vi "Dashboard Main.vi"() -> ()   [LabVIEW 2018]
uses:
  <vilib>/Utility/miscctls.llb/LVRowAndColumnTypeDef.ctl
  <vilib>/event_ctls.llb/eventvkey.ctl
  <vilib>/Rock Robotics/Network Tables/NT Read Numeric Array.vi
  <vilib>/Rock Robotics/Network Tables/NT Write Boolean.vi
  <vilib>/Rock Robotics/WPI/Dashboard/WPI_DashboardLogging Global.vi
panel:
  in  "Camera Settings Right":T1={"Frame Rate"=30, "Compression"=30, "Size"=1, "DB Camera Config"=FALSE} {"Frame Rate" scale=1.0..30.0; "Compression" scale=100.0..-1.0; "Size" items=["640x480", "320x240", "160x120"]}
  in  "Camera Name Right":string(combo)="No Camera Selection"
  out "Camera Perf":string
  in  "Camera Settings":T1={"Frame Rate"=30, "Compression"=30, "Size"=1, "DB Camera Config"=FALSE} {"Frame Rate" scale=1.0..30.0; "Compression" scale=100.0..-1.0; "Size" items=["640x480", "320x240", "160x120"]}
  in  "TCP":refnum<k5>
  in  "Rec Mode":enum32{"Stop", "Record", "Playback"}(radio)
  out "Robot IP":string
  out "Image Message":string="Timeout in Camera Communications"
  in  "Dashboard Tab":T2(tab)
  in  "Select Auto":string(combo)="Select Autonomous ..."
  out "NT Connection":bool
  out "MotorChart R":cluster{"Numeric":dbl, "Numeric":dbl}(graph)
  out "MotorChart L":cluster{"Numeric":dbl, "Numeric":dbl}(graph)
  out "MotorSliders R":cluster{"MotorSlide1":dbl, "MotorSlide2":dbl} {"MotorSlide2" scale=-1.0..1.0 scale format="%#_2e"; "MotorSlide1" scale=-1.0..1.0 scale format="%#_2e"}
  out "MotorSliders L":cluster{"MotorSlide1":dbl, "MotorSlide2":dbl} {"MotorSlide2" scale=-1.0..1.0 scale format="%#_2e"; "MotorSlide1" scale=-1.0..1.0 scale format="%#_2e"}
  out "Gyro":dbl(knob) scale=0.0..360.0
  out "JS1 Z":dbl(slide) scale=-1.0..1.0 scale format="%#_2e"
  out "JS1 Graph":cluster{"X":dbl, "Y":dbl}[](graph)
  out "JS1 Buttons":T3
  out "JS2 Z":dbl(slide) scale=-1.0..1.0 scale format="%#_2e"
  out "JS2 Graph":cluster{"X":dbl, "Y":dbl}[](graph)
  out "JS2 Buttons":T3
  out "Mode":T4(ring)=enum."Auto Disabled"
  out "Right Camera Perf":cluster{"Bandwidth (Mbps)":dbl, "FPS":dbl}
  out "Camera Image Right":T5(plugin-control)
  in  "DB/String 9":string
  in  "DB/String 8":string
  in  "DB/String 7":string
  in  "DB/String 6":string
  in  "DB/String 5":string
  in  "DB/String 4":string
  in  "DB/String 3":string
  in  "DB/String 2":string
  in  "DB/String 1":string
  in  "DB/String 0":string
  in  "DB/Slider 0":dbl(slide) scale=0.0..5.0
  in  "DB/Slider 1":dbl(slide) scale=0.0..5.0
  in  "DB/Slider 2":dbl(slide) scale=0.0..5.0
  in  "DB/Slider 3":dbl(slide) scale=0.0..5.0
  out "DB/LED 3":bool
  out "DB/LED 2":bool
  out "DB/LED 1":bool
  out "DB/LED 0":bool
  in  "DB/Button 3":bool
  in  "DB/Button 2":bool
  in  "DB/Button 1":bool
  in  "DB/Button 0":bool caption="New Name"
  in  "Mode":T6(ring)
  in  "Zero Horse Encoder":bool
  in  "Zero Elevator Encoder":bool
  in  "Zero Wrist Encoder":bool
  in  "Place Level 3":bool
  in  "Place Level 2":bool
  in  "Place Level 1":bool
  in  "Cargo Ship":bool
  in  "Intake Feeder":bool
  in  "Intake Ground":bool
  in  "Elevator Control":dbl(slide) step=0.05 scale=-1.0..1.0
  in  "Wrist Control":dbl(slide) step=0.05 scale=-1.0..1.0
  in  "Test Slider":dbl(slide) scale=0.0..100.0 scale format="%#_3g"
  in  "On/Off":bool caption="Solenoid"
  in  "Test Name":u16(ring) items=["Select the test to run..."]
  in  "Test Tree":string(tree)
  in  "Motor":cluster{"Value":dbl, "Enable":bool} {"Value" scale=-1.0..1.0 scale format="%#_3g"}
  out "Progress":T7 {"Test Progress" scale=0.0..100.0}
  in  "Rev/Fwd":cluster{"Forward":bool, "Reverse":bool}
  in  "Test Ring":u16(ring) items=["Monochrome", "Color"]
  out "Cmd Status":string
  in  "Execute Command":bool
  in  "Command Params":string[][](table)
  in  "Command Selection":i32(listbox)
  in  "CheckList":i32(listbox)
  out "Tree":string(tree)
  out "Camera Image":T5(plugin-control)
  out "Background":bool
  in  "Camera Name":string(combo)="No Camera Selection"
  # "HW"
  # "HW"
  # "Joysticks"
  # "Drive Motors"
  # "Front"
  # "Right"
  # "Left"
  # "Back"
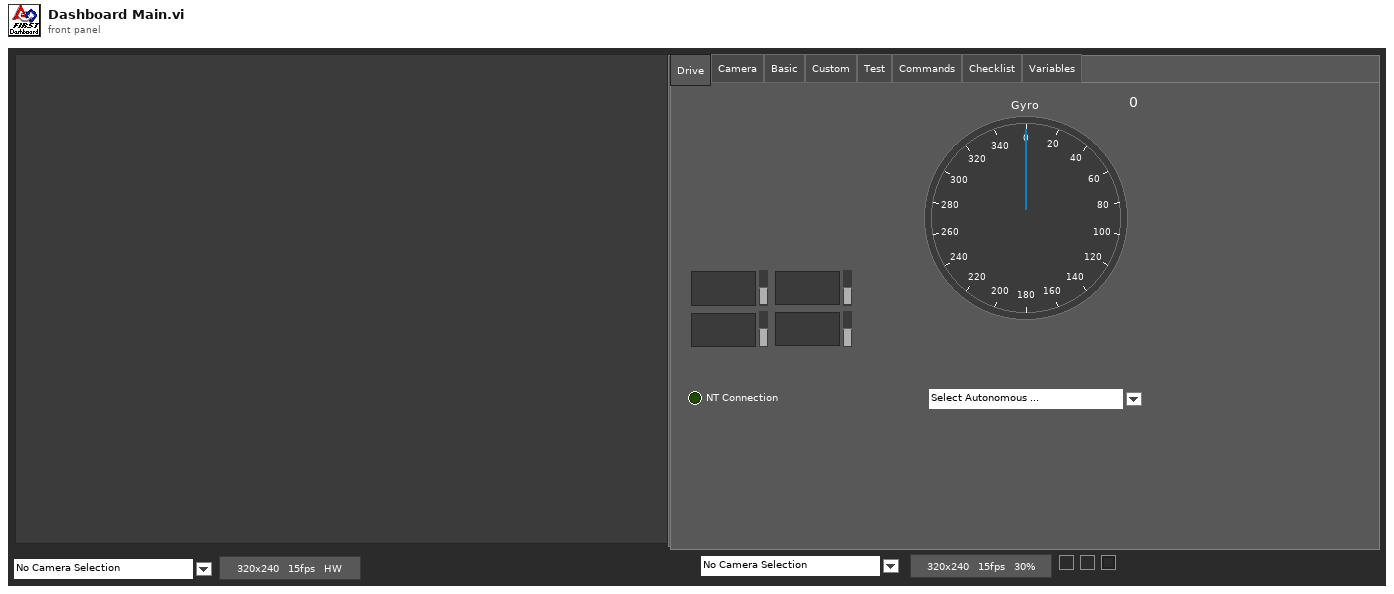
[diagram p1: front panel]
types:
  T1 = cluster{"Frame Rate":i32, "Compression":i32, "Size":u16, "DB Camera Config":bool}
  T2 = enum32{"Drive", "Camera", "Basic", "Custom", "Test", "Commands", "Checklist", "Variables"}
  T3 = cluster{bool, bool, bool, bool, bool, bool, bool, bool, bool, bool, bool, bool}
  T4 = enum8{"Tele-Op Disabled", "Tele-Op Enabled", "Auto Disabled", "Auto Enabled", "Test Disabled", "Test Enabled", "Disconnected", "No Code", "E-Stop"}
  T5 = typedef "IMAQ Image.ctl" = refnum<image>
  T6 = enum16{"Operator Console", "Hatch", "Cargo", "Horse Hatch", "Override to Manual"}
  T7 = cluster{"Test Progress":u8, "Test Progress Text":string}
  T8 = cluster{"Save Path":path, "Interval (s)":dbl, "Keep":i32}
  T9 = typedef "Image Type" = u32
  T10 = cluster{"IDs":cluster{"RPC field ID":u16, "Unique ID":u16}, "String":string}
  T11 = cluster{"Error Strings":string, "Disable Counts":cluster{u16, u16}, "Rail Faults":cluster{u16, u16, u16}, "Robot IP":string, "DB Mode":u8, "Event Info":cluster{"Name":string, "Type":u8, "Number":u16, "Replay":u8}}
  T12 = cluster{"Storage":cluster{"Disk Free":u64, "RAM Block":u32, "RAM free":u32}, "CPU Utilization":cluster{"CPU % ISR":sgl, "CPU % Time Crit":sgl, "CPU % Timed Str":sgl, "CPU % High":sgl, "CPU % Above":sgl, "CPU % Normal":sgl, "CPU % Low":sgl}, "CAN":cluster{"% Bus Utilization":sgl, "Bus Off Cnt":u32, "TX_FIFO Full Cnt":u32, "Receive Error Cnt":u8, "Transmit Error Cnt":u8}, "HID":cluster{"HID Outputs":u32, "Rumble Low":u16, "Rumble High":u16}[]}
  T13 = cluster{"Status bits":cluster{"Test Mode":bool, "Autonomous":bool, "Enabled":bool, "Code Start":bool, "Brownout":bool, "Reserved 2":bool, "Reserved 3":bool, "E-Stop":bool}, "Code Trace":cluster{"Disabled":bool, "TeleOp":bool, "Auto":bool, "Test":bool}, "Controller Type":enum16{"unknown", "cRIO", "roboRio"}, "Code?":enum16{"unknown", "noCode", "code"}, "Battery V":dbl}
  T14 = cluster{"Control Bits":cluster{"TestMode":bool, "Autonomous":bool, "Enabled":bool, "FMS Present":bool, bool, bool, bool, "E-Stop":bool}, "Team Station ":u8, "Countdown":sgl, "Joystick Values":cluster{"Axes":dbl[], "Buttons":bool[], "POVs":i16[]}[]}
  T15 = cluster{"Axes":dbl[], "Buttons":bool[], "POVs":i16[]}[]
  T16 = cluster{"Axes":dbl[], "Buttons":bool[], "POVs":i16[]}
  T17 = cluster{"Buttons[0]":bool, "Buttons[1]":bool, "Buttons[2]":bool, "Buttons[3]":bool, "Buttons[4]":bool, "Buttons[5]":bool, "Buttons[6]":bool, "Buttons[7]":bool, "Buttons[8]":bool, "Buttons[9]":bool, "Buttons[10]":bool, "Buttons[11]":bool}
  T18 = cluster{"Camera Image":refnum<vi>, "Dashboard Tab":refnum<vi>, "Background":refnum<vi>, "Rec Mode":refnum<vi>, "Test Slider":refnum<vi>, "On/Off ":refnum<vi>, "Test Ring":refnum<vi>, "Rev/Fwd":refnum<vi>, "Test Name":refnum<vi>, "Motor":refnum<vi>, "Progress":refnum<vi>, "CheckList":refnum<vi>, "Tree":refnum<vi>, "Test Tree":refnum<vi>, "Command Params":refnum<vi>, "Command Selection":refnum<vi>, "Execute Command":refnum<vi>, "Cmd Status":refnum<vi>, "Camera Settings":refnum<vi>, "Camera Name":refnum<vi>, "Camera Perf":refnum<vi>, "Camera Settings Right":refnum<vi>, "Camera Name Right":refnum<vi>, "Camera Image Right":refnum<vi>}
  T19 = cluster{"Global Rectangle":i32[], "Contours":cluster{"Contour Type":u32, "ROI Type":u32, "Points":i32[]}[]}
  T20 = cluster{"Camera Name":string, string, "Saved DB Images Info":cluster{"Save Path":path, "Interval (s)":dbl, "Keep":i32}}
  T21 = cluster{"Camera Name Right":string, string, "Saved DB Images Info":cluster{"Save Path":path, "Interval (s)":dbl, "Keep":i32}}
  T22 = cluster{"Operation":enum16{"Update", "Clear"}, "Color Box":u32}[]
  T23 = typedef "eventvkey.ctl" = enum16{"ASCII", "Enter", "Return", "Shift", "Ctrl", "Alt", "Cmd", "Opt", "Caps", "NumLock", "Clear", "Break", "Up", "Down", "Left", "Right", "Insert", "Delete", "Home", "End", "PageUp", "PageDown", "Escape", "Help", "Pause", "ScrollLock", "F1", "F2", "F3", "F4", "F5", "F6", "F7", "F8", "F9", "F10", "F11", "F12", "F13", "F14", "F15", "F16", "F17", "F18", "F19", "F20", "F21", "F22", "F23", "F24", "Play", "VolumeUp", "VolumeDown", "Mute", "Two Byte Char"}
  T24 = cluster{"Image Size":bool, "Image Type":bool, "Pixel Value":bool, "ROI Information":bool, "Zoom Factor":bool}
  T25 = cluster{"Operation":enum16{"Update", "Clear"}, "Color Box":u32}
  T26 = typedef "LVRowAndColumnTypeDef.ctl" = cluster{"Row":i32, "Column":i32}
  T27 = cluster{"Shift":bool, "Ctrl":bool, "Alt":bool, "Cmd":bool, "Opt":bool}
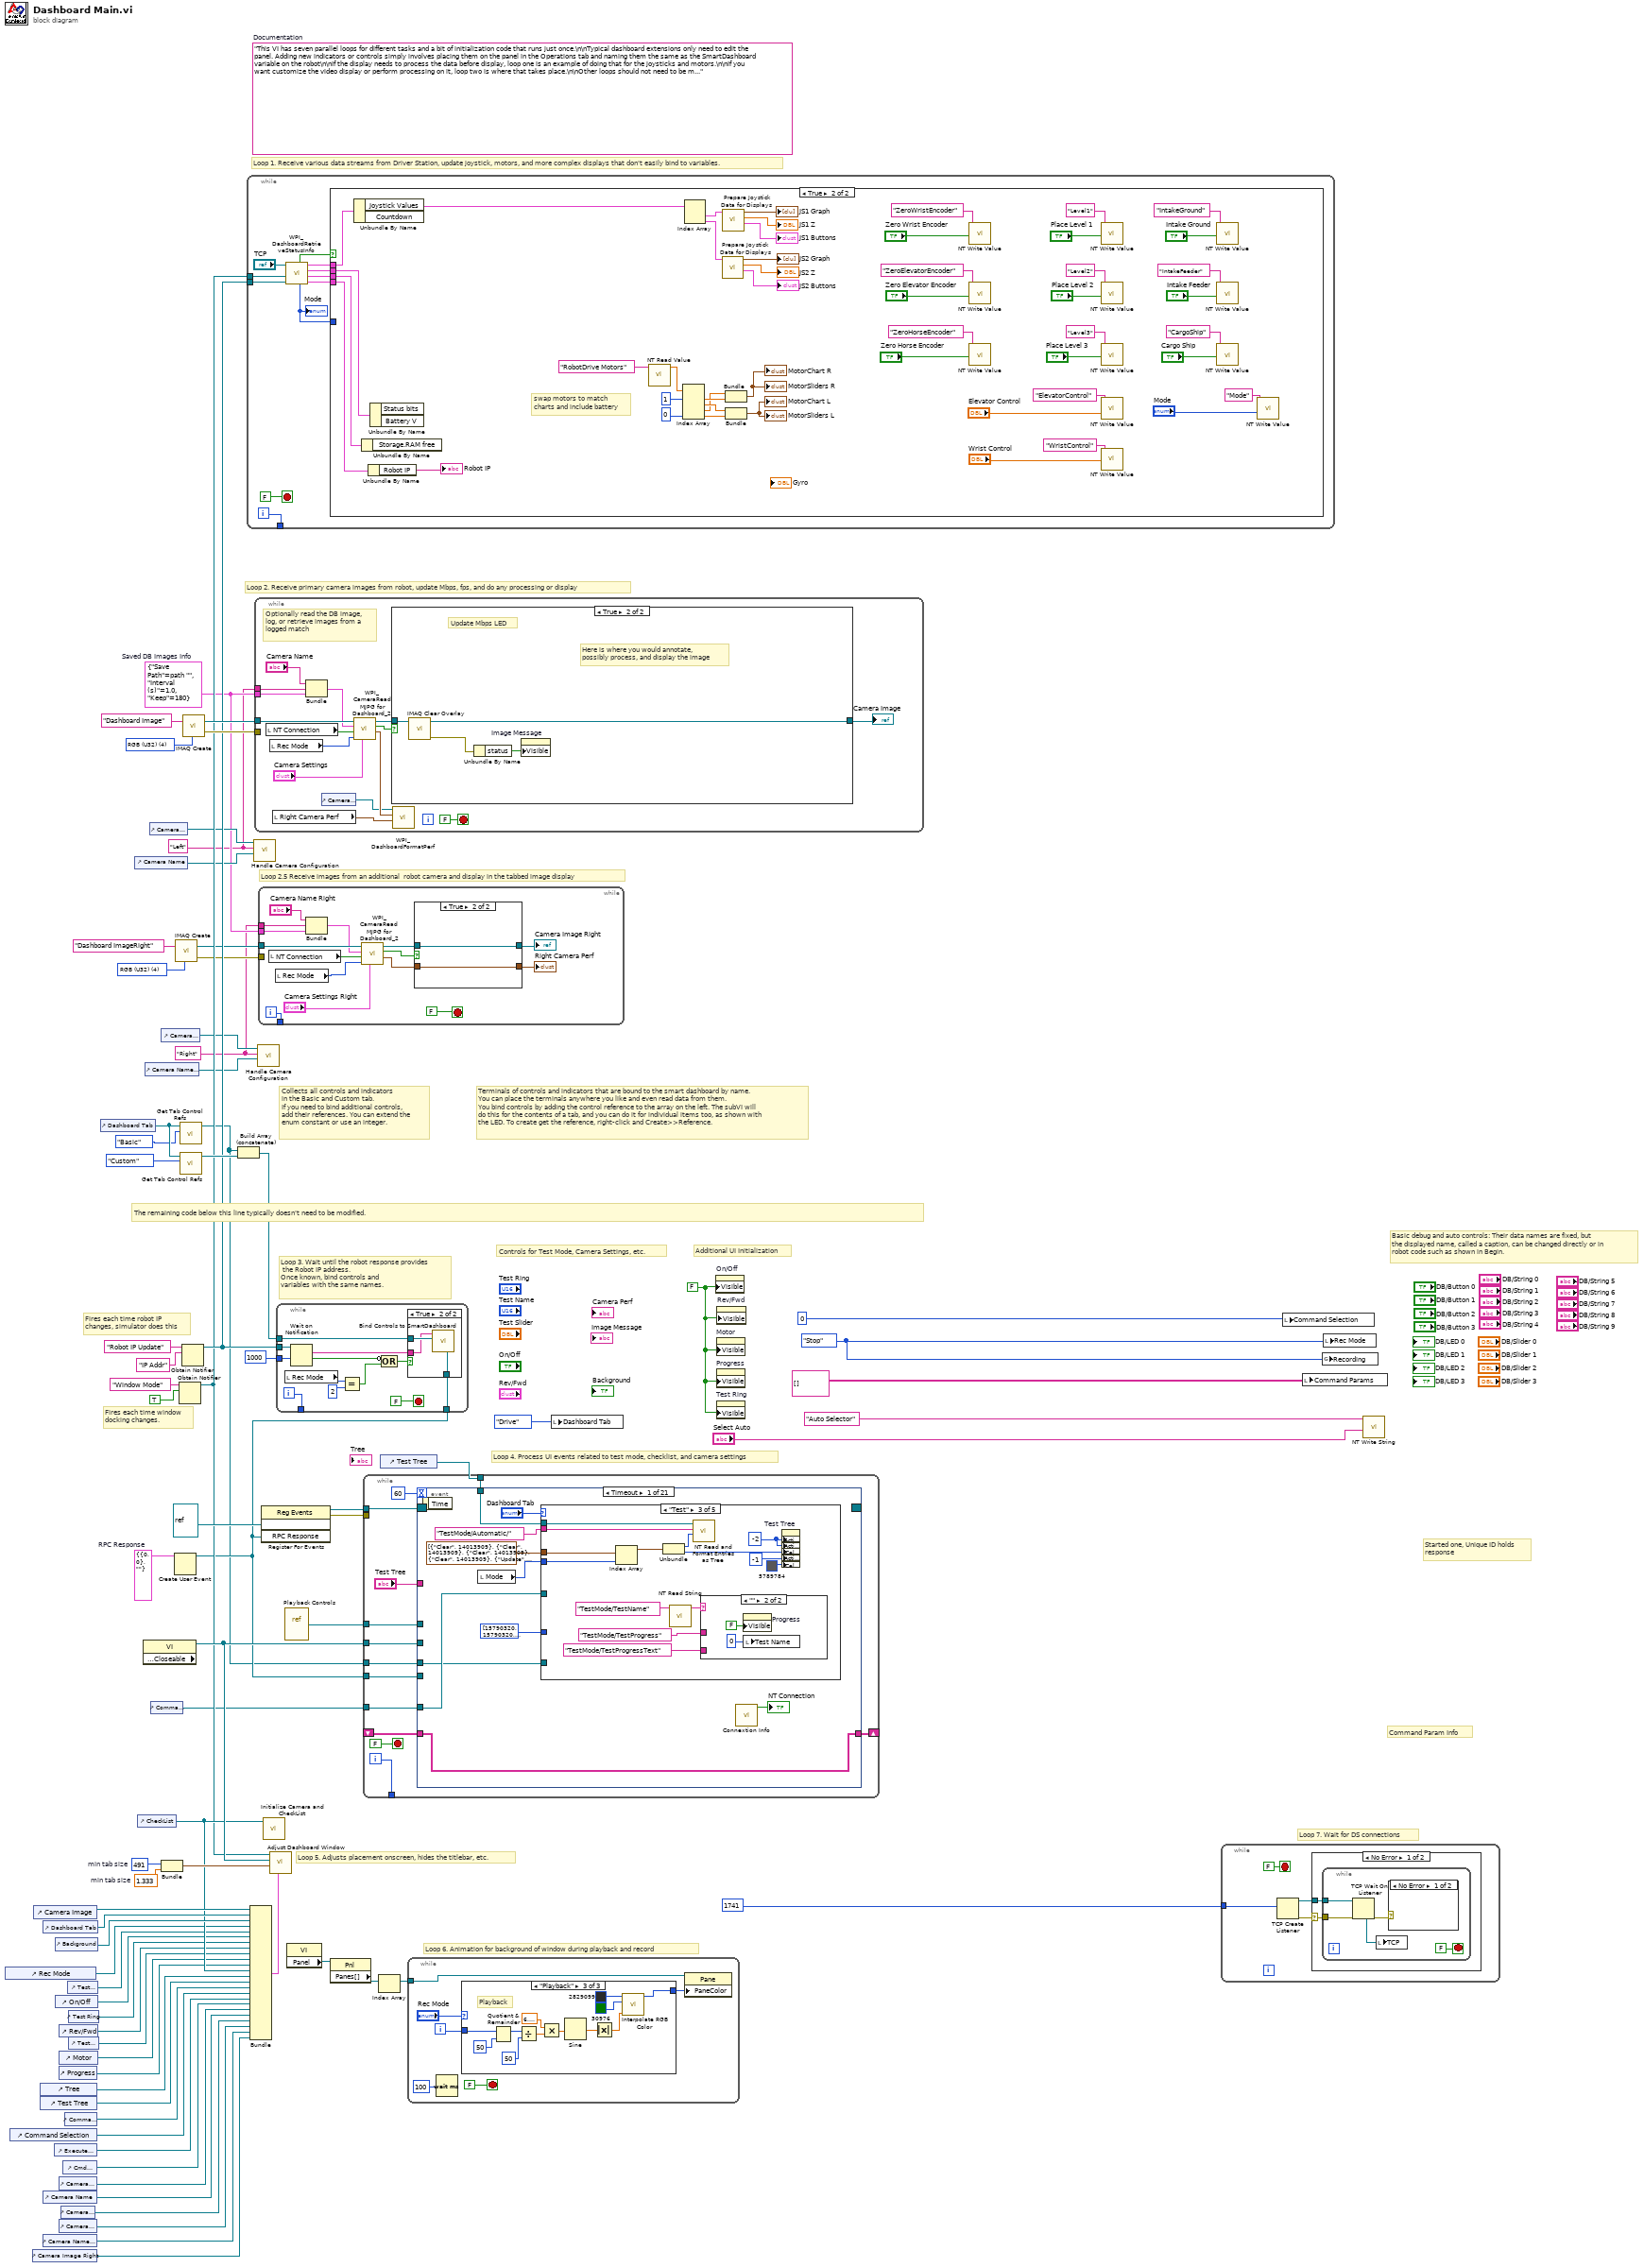
[diagram p0: block diagram]
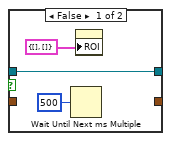
[diagram p2: hidden frame]
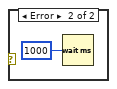
[diagram p3: hidden frame]
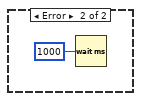
[diagram p4: hidden frame]
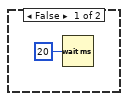
[diagram p5: hidden frame]
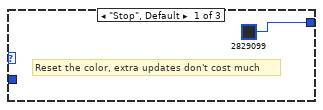
[diagram p6: hidden frame]
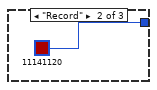
[diagram p7: hidden frame]
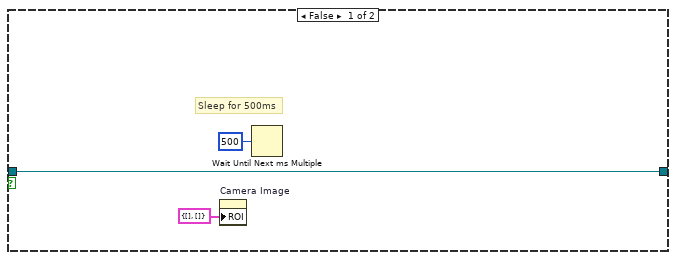
[diagram p9: hidden frame]
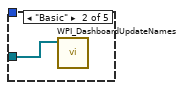
[diagram p11: hidden frame]
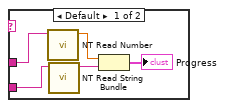
[diagram p12: hidden frame]
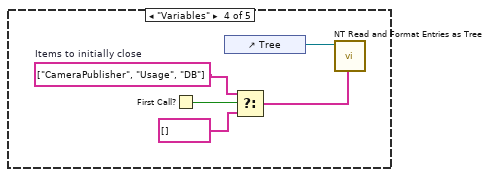
[diagram p13: hidden frame]
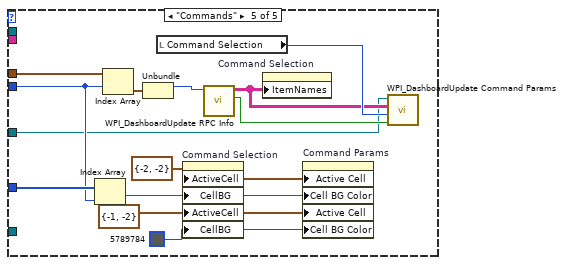
[diagram p14: hidden frame]
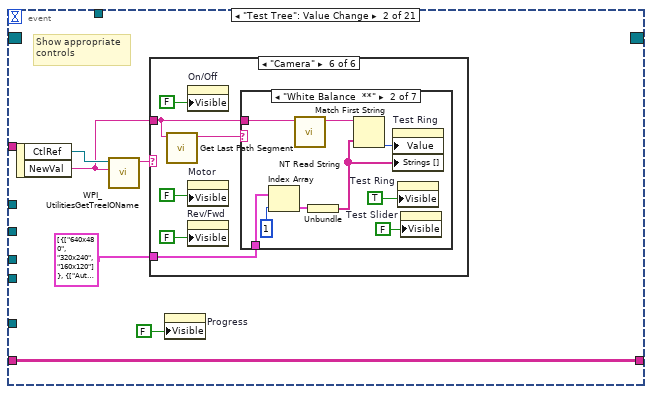
[diagram p15: hidden frame]
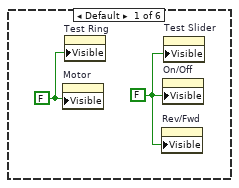
[diagram p16: hidden frame]
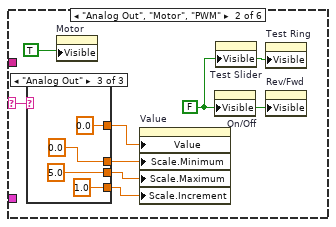
[diagram p17: hidden frame]
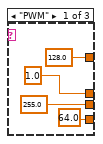
[diagram p18: hidden frame]
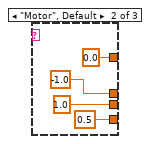
[diagram p19: hidden frame]
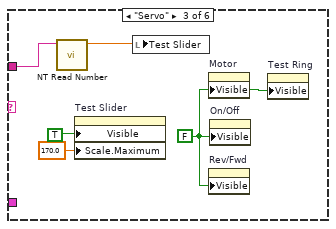
[diagram p20: hidden frame]
diagram:
  w3 = T8 {"Save Path"=path "", "Interval (s)"=1.0, "Keep"=180}  # Saved DB Images Info
  w2 = "Right"
  w1 = "Left"
  w13 = T9 4 items=["Grayscale (U8)", "Grayscale (I16)", "Grayscale (SGL)", "Complex (CSG)", "RGB (U32)", "HSL (U32)", "RGB (U64)"] ("Image Type")
  w29 = T10 {"IDs"={"RPC field ID"=0, "Unique ID"=0}, "String"=""}  # RPC Response
  w52 = 491  # min tab size
  w51 = 1.333  # min tab size
  w59 = enum32{"Stop", "Record", "Playback"}."Stop" ("Rec Mode")
  w36 = FALSE ("Visible")
  (unwired) "This VI has seven parallel loops for different tasks and a bit of initialization code that runs just once.\n\nTypical dashboard extensions only need to edit the panel. Adding new indicators or controls simply involves placing them on the panel in the Operations tab and naming them the same as the SmartDashboard variable on the robot\n\nIf the display needs to process the data before display, loop one is an example of doing that for the joysticks and motors.\n\nIf you want customize the video display or perform processing on it, loop two is where that takes place.\n\nOther loops should not need to be modified. They are pretty standard, and document the task they perform."  # Documentation
  w76 = T9 4 items=["Grayscale (U8)", "Grayscale (I16)", "Grayscale (SGL)", "Complex (CSG)", "RGB (U32)", "HSL (U32)", "RGB (U64)"] ("Image Type")
  # "Loop 2.5 Receive images from an additional  robot camera and display in the tabbed image display"
  # "Command Param Info"
  # "Started one, Unique ID holds\nresponse"
  # "Loop 7. Wait for DS connections"
  # "Basic debug and auto controls: Their data names are fixed, but\nthe displayed name, called a caption, can be changed directly or in\nrobot code such as shown in Begin."
  # "Controls for Test Mode, Camera Settings, etc."
  # "Additional UI Initialization"
  # "Loop 6. Animation for background of window during playback and record"
  # "Fires each time robot IP\nchanges, simulator does this"
  # "Fires each time window\ndocking changes."
  # "Collects all controls and indicators\nin the Basic and Custom tab.\nIf you need to bind additional controls,\nadd their references. You can extend the\nenum constant or use an integer."
  # "The remaining code below this line typically doesn't need to be modified."
  # "Loop 4. Process UI events related to test mode, checklist, and camera settings"
  # "Terminals of controls and indicators that are bound to the smart dashboard by name.\nYou can place the terminals anywhere you like and even read data from them.\nYou bind controls by adding the control reference to the array on the left. The subVI will\ndo this for the contents of a tab, and you can do it for individual items too, as shown with\nthe LED. To create get the reference, right-click and Create>>Reference."
  # "Loop 3. Wait until the robot response provides\n the Robot IP address.\nOnce known, bind controls and\nvariables with the same names."
  # "Loop 5. Adjusts placement onscreen, hides the titlebar, etc."
  # "Loop 1. Receive various data streams from Driver Station, update joystick, motors, and more complex displays that don't easily bind to variables."
  # "Loop 2. Receive primary camera images from robot, update Mbps, fps, and do any processing or display"
  n1 = control-ref of="Rec Mode"() -> (w42:refnum<vi>)
  n2 = control-ref of="Command Selection"() -> (w28:refnum<vi>)
  n3 = control-ref of="Camera Image Right"() -> (w6:refnum<vi>)
  n4 = control-ref of="Camera Image"() -> (w54:refnum<vi>)
  n5 = control-ref of="Tree"() -> (w46:refnum<vi>)
  n6 = control-ref of="Test Tree"() -> (w45:refnum<vi>)
  n7 = control-ref of="Dashboard Tab"() -> (w53:refnum<vi>)
  n8 = control-ref of="Camera Name"() -> (w19:refnum<vi>)
  n9 = control-ref of="Camera Name Right"() -> (w7:refnum<vi>)
  n10 = control-ref of="Execute Command"() -> (w30:refnum<vi>)
  n11 = control-ref of="Background"() -> (w49:refnum<vi>)
  n12 = control-ref of="On/Off"() -> (w40:refnum<vi>)
  n13 = control-ref of="Progress"() -> (w37:refnum<vi>)
  n14 = control-ref of="Camera Settings"() -> (w20:refnum<vi>)
  n15 = control-ref of="Camera Settings Right"() -> (w8:refnum<vi>)
  n16 = control-ref of="Rev/Fwd"() -> (w38:refnum<vi>)
  n17 = control-ref of="Motor"() -> (w43:refnum<vi>)
  n18 = control-ref of="Camera Perf"() -> (w18:refnum<vi>)
  n19 = control-ref of="Cmd Status"() -> (w24:refnum<vi>)
  n20 = control-ref of="Command Params"() -> (w31:refnum<vi>)
  n21 = control-ref of="Test Slider"() -> (w41:refnum<vi>)
  n22 = control-ref of="Test Ring"() -> (w39:refnum<vi>)
  n23 = control-ref of="Test Name"() -> (w44:refnum<vi>)
  n24 = control-ref of="Dashboard Tab"() -> (w57:refnum<vi>)
  n25 = control-ref of="Camera Name"() -> (w21:refnum<vi>)
  n26 = control-ref of="CheckList"() -> (w47:refnum<vi>)
  n27 = property class="VI" props=["Front Panel.Closeable"]() -> (reference out=w58:refnum<vi>)  [unwired: 2 in, 2 out]
  n28 = control-ref of="Camera Name Right"() -> (w9:refnum<vi>)
  n29 = control-ref of="Camera Settings"() -> (w22:refnum<vi>)
  n30 = control-ref of="Command Params"() -> (w23:refnum<vi>)
  n31 = control-ref of="Camera Settings Right"() -> (w10:refnum<vi>)
  n32 = Bundle("min tab size"=w52, "min tab size"=w51) -> (w50:cluster{"min tab size":i32, "min tab size":dbl})  [unwired: 1 in]
  n33 = Create User Event(user event datatype=w29) -> (user event=w25:refnum<user-event>)  [unwired: 1 in, 1 out]
  n34 = call "IMAQ Create"("Image Name"="Dashboard ImageRight", "Image Type"=w13) -> ("New Image"=w12:T5, "error out"=w11:errorcluster)  [unwired: 2 in, 1 out]
  n35 = Obtain Notifier(name (unnamed)="Window Mode", notification data type=TRUE) -> (notifier out=w34:refnum<notifier>)  [unwired: 2 in, 2 out]
  n36 = call <vilib>:"Get Tab Control Refs.vi"("Page Index"=T2."Basic" ("Dashboard Tab"), "TabControl in"=w57) -> ("ControlsOnPage"=w17:refnum<vi>[])  [unwired: 9 in]
  n37 = call <vilib>:"Get Tab Control Refs.vi"("Page Index"=T2."Custom" ("Dashboard Tab"), "TabControl in"=w57) -> ("ControlsOnPage"=w56:refnum<vi>[])  [unwired: 9 in]
  n38 = Obtain Notifier(name (unnamed)="Robot IP Update", notification data type="IP Addr" ("name (unnamed)")) -> (notifier out=w35:refnum<notifier>)  [unwired: 2 in, 2 out]
  n39 = call "IMAQ Create"("Image Name"="Dashboard Image", "Image Type"=w76) -> ("New Image"=w74:T5, "error out"=w73:errorcluster)  [unwired: 2 in, 1 out]
  n40 = Build Array (concatenate)(w17, w56) -> (w55:refnum<vi>[])
  n41 = while {
    tunnel: [w86] -> _
    tunnel: w35 -> [w80]
    tunnel: w34 -> [w77]
    i -> [w86]
    stop <- FALSE stop-if-true
    n42 = call <vilib>:"WPI_DashboardRetrieveStatusInfo.vi"("Binding Refnum"=w80, "Window Mode Notifier"=w77, "TCP Cnx"="TCP") -> ("Power and Errors"=w81:T11, "Robot Metrics"=w84:T12, "Status Info"=w85:T13, "Control Info"=w82:T14, "Robot Mode"=w79:T4, "Process?"=w83:bool)  [unwired: 3 in]
    "Mode" <- w79
    n43 = case shown="True" w83 {
      tunnel: w85 -> [_ w136]
      tunnel: w84 -> [_ w135]
      tunnel: w82 -> [_ w134]
      tunnel: w81 -> [_ w133]
      tunnel: w79 -> [_ _]
      frame False {
        n44 = Wait (ms)(milliseconds to wait=u32 20) -> ()  [unwired: 1 out]
      }
      frame True {
        # "swap motors to match\ncharts and include battery"
        n45 = Unbundle By Name(w134) -> ("Joystick Values"=w124:T15)  [unwired: 1 out]
        n46 = Unbundle By Name(w135) -> ()  [unwired: 1 out]
        n47 = Unbundle By Name(w133) -> ("Robot IP"=→"Robot IP":string)
        n48 = Unbundle By Name(w136) -> ()  [unwired: 2 out]
        n49 = call-poly <vilib>:"NT Read Value.vi"("Name"="RobotDrive Motors") -> ("Numeric Array"=w114:dbl[])  [unwired: 9 in, 1 out]
        n50 = Index Array(array=w114, index #1=1, index #4=0) -> (element #1=w128:dbl, element #2=w129:dbl, element #3=w127:dbl, element #4=w132:dbl)  [unwired: 2 in]
        n51 = Index Array(array=w124) -> (element #1=w123:T16, element #2=w119:T16)  [unwired: 2 in]
        n52 = call "Prepare Joystick Data for Displays.vi"("Joystick Values"=w119) -> ("Buttons"=→"JS2 Buttons":T17, "Z Axis"=→"JS2 Z":dbl, "Cartesian Data"=→"JS2 Graph":cluster{"X axis":dbl, "X axis":dbl}[])  [unwired: 8 in]
        n53 = call "Prepare Joystick Data for Displays.vi"("Joystick Values"=w123) -> ("Buttons"=→"JS1 Buttons":T17, "Z Axis"=→"JS1 Z":dbl, "Cartesian Data"=→"JS1 Graph":cluster{"X axis":dbl, "X axis":dbl}[])  [unwired: 8 in]
        n54 = Bundle("Numeric"=w127, "Numeric"=w128) -> (→"MotorChart R" →"MotorSliders R":cluster{"Numeric":dbl, "Numeric":dbl})  [unwired: 1 in]
        n55 = Bundle("Numeric"=w129, "Numeric"=w132) -> (→"MotorChart L" →"MotorSliders L":cluster{"Numeric":dbl, "Numeric":dbl})  [unwired: 1 in]
        n56 = call-poly <vilib>:"NT Write Value.vi"("Boolean"="Zero Wrist Encoder", "Name"="ZeroWristEncoder") -> ()  [unwired: 9 in, 1 out]
        n57 = call-poly <vilib>:"NT Write Value.vi"("Boolean"="Zero Elevator Encoder", "Name"="ZeroElevatorEncoder") -> ()  [unwired: 9 in, 1 out]
        n58 = call-poly <vilib>:"NT Write Value.vi"("Boolean"="Zero Horse Encoder", "Name"="ZeroHorseEncoder") -> ()  [unwired: 9 in, 1 out]
        n59 = call-poly <vilib>:"NT Write Value.vi"("Boolean"="Place Level 1", "Name"="Level1") -> ()  [unwired: 9 in, 1 out]
        n60 = call-poly <vilib>:"NT Write Value.vi"("Boolean"="Place Level 2", "Name"="Level2") -> ()  [unwired: 9 in, 1 out]
        n61 = call-poly <vilib>:"NT Write Value.vi"("Boolean"="Place Level 3", "Name"="Level3") -> ()  [unwired: 9 in, 1 out]
        n62 = call-poly <vilib>:"NT Write Value.vi"("Numeric"="Elevator Control", "Name"="ElevatorControl") -> ()  [unwired: 9 in, 1 out]
        n63 = call-poly <vilib>:"NT Write Value.vi"("Numeric"="Wrist Control", "Name"="WristControl") -> ()  [unwired: 9 in, 1 out]
        n64 = call-poly <vilib>:"NT Write Value.vi"("Boolean"="Intake Ground", "Name"="IntakeGround") -> ()  [unwired: 9 in, 1 out]
        n65 = call-poly <vilib>:"NT Write Value.vi"("Boolean"="Intake Feeder", "Name"="IntakeFeeder") -> ()  [unwired: 9 in, 1 out]
        n66 = call-poly <vilib>:"NT Write Value.vi"("Boolean"="Cargo Ship", "Name"="CargoShip") -> ()  [unwired: 9 in, 1 out]
        n67 = call-poly <vilib>:"NT Write Value.vi"("Numeric"="Mode", "Name"="Mode") -> ()  [unwired: 9 in, 1 out]
      }
    }
  }
  n68 = Bundle("Camera Image"=w54, "Dashboard Tab"=w53, "Background"=w49, "Rec Mode"=w42, "Test Slider"=w41, "On/Off"=w40, "Test Ring"=w39, "Rev/Fwd"=w38, "Test Name"=w44, "Motor"=w43, "Progress"=w37, "CheckList"=w47, "Tree"=w46, "Test Tree"=w45, "Command Params"=w31, "Command Selection"=w28, "Execute Command"=w30, "Cmd Status"=w24, "Camera Settings"=w20, "Camera Name"=w19, "Camera Perf"=w18, "Camera Settings Right"=w8, "Camera Name Right"=w7, "Camera Image Right"=w6) -> (w48:T18)  [unwired: 1 in]
  n69 = call "Handle Camera Configuration.vi"("CameraNameRef"=w21, "Display Name"=w1, "ClusterRef"=w22) -> ()  [unwired: 9 in]
  n70 = while {
    tunnel: w74 -> [w150]
    tunnel: w73 -> [_]
    tunnel: w3 -> [w143]
    tunnel: w1 -> [w140]
    stop <- FALSE stop-if-true
    # "Optionally read the DB image,\nlog, or retrieve images from a\nlogged match"
    n71 = local read "NT Connection"() -> (w144:bool)
    n72 = local read "Rec Mode"() -> (w147:enum32{"Stop", "Record", "Playback"})
    n73 = local read "Right Camera Perf"() -> (w138:cluster{"Bandwidth (Mbps)":dbl, "FPS":dbl})
    n74 = Bundle("Camera Name"="Camera Name", w140, "Saved DB Images Info"=w143) -> (w142:T20)  [unwired: 1 in]
    n75 = control-ref of="Camera Perf"() -> (w137:refnum<vi>)
    n76 = call <vilib>:"WPI_CameraRead MJPG for Dashboard_2.vi"("Camera Settings"="Camera Settings", "Rec Mode"=w147, "NT Connection"=w144, "Capture Info"=w142, "Image in"=w150) -> ("perf info"=w139:cluster{"Bandwidth (Mbps)":dbl, "fps":dbl}, "Active"=w148:bool, "Image\\ out"=w149:T5)  [unwired: 4 in]
    n77 = case shown="True" w148 {
      tunnel: w149 -> [w153 w156]
      tunnel: [w153 w155] -> w145
      frame False {
        # "Sleep for 500ms"
        n78 = property on="Camera Image" class="ImageControl"("ROI"=T19 {"Global Rectangle"=[], "Contours"=[]}) -> ()  [unwired: 2 in, 2 out]
        n79 = Wait Until Next ms Multiple(millisecond multiple=u32 500) -> ()  [unwired: 1 out]
      }
      frame True {
        # "Here is where you would annotate,\npossibly process, and display the image"
        # "Update Mbps LED"
        n80 = call "IMAQ Clear Overlay"("Image"=w156) -> ("error out"=w157:errorcluster, "Image Out"=w155:T5)  [unwired: 2 in, 7 out]
        n81 = Unbundle By Name(w157) -> ("status"=w158:bool)
        n82 = property on="Image Message" class="Str"("Visible"=w158) -> ()  [unwired: 2 in, 2 out]
      }
    }
    "Camera Image" <- w145
    n83 = call <vilib>:"WPI_DashboardFormatPerf.vi"("Right Camera Perf"=w138, "Performance"=w139, "String in"=w137) -> ()  [unwired: 9 in]
  }
  n84 = call "Handle Camera Configuration.vi"("CameraNameRef"=w9, "Display Name"=w2, "ClusterRef"=w10) -> ()  [unwired: 9 in]
  n85 = while {
    tunnel: w12 -> [w173]
    tunnel: w11 -> [_]
    tunnel: [w168] -> _
    tunnel: w3 -> [w164]
    tunnel: w2 -> [w161]
    i -> [w168]
    stop <- FALSE stop-if-true
    n86 = local read "NT Connection"() -> (w165:bool)
    n87 = local read "Rec Mode"() -> (w172:enum32{"Stop", "Record", "Playback"})
    n88 = Bundle("Camera Name Right"="Camera Name Right", w161, "Saved DB Images Info"=w164) -> (w163:T21)  [unwired: 1 in]
    n89 = call <vilib>:"WPI_CameraRead MJPG for Dashboard_2.vi"("Camera Settings"="Camera Settings Right", "Rec Mode"=w172, "NT Connection"=w165, "Capture Info"=w163, "Image in"=w173) -> ("perf info"=w159:cluster{"Bandwidth (Mbps)":dbl, "fps":dbl}, "Active"=w167:bool, "Image\\ out"=w170:T5)  [unwired: 4 in]
    n90 = case shown="True" w167 {
      tunnel: w170 -> [w175 w178]
      tunnel: [w175 w178] -> w166
      tunnel: [_ w177] -> w160
      tunnel: w159 -> [_ w177]
      frame False {
        n91 = Wait Until Next ms Multiple(millisecond multiple=u32 500) -> ()  [unwired: 1 out]
        n92 = property on="Camera Image Right" class="ImageControl"("ROI"=T19 {"Global Rectangle"=[], "Contours"=[]}) -> ()  [unwired: 2 in, 2 out]
      }
      frame True {
      }
    }
    "Camera Image Right" <- w166
    "Right Camera Perf" <- w160
  }
  n93 = register-events(refnum<vi> refnum, w25) -> (reference out=w63:refnum<event-registration>, error out=w62:errorcluster)  [unwired: 2 in]
  n94 = call "Initialize Camera and CheckList.vi"("ListBox in"=w47) -> ()  [unwired: 11 in]
  n95 = call "Adjust Dashboard Window.vi"("Sizing Refnums"=w48, "Size Constraints"=w50, "VI"=w58, "WIn Mode"=w34) -> ()  [unwired: 8 in]
  n96 = while {
    tunnel: w55 -> [w190]
    tunnel: w35 -> [w188]
    tunnel: [w186] -> _
    tunnel: u32 1000 ("milliseconds to wait") -> [w185]
    tunnel: w25 -> [w179]
    i -> [w186]
    stop <- FALSE stop-if-true
    n97 = local read "Rec Mode"() -> (w181:enum32{"Stop", "Record", "Playback"})
    n98 = Wait on Notification(notifier=w188, timeout in ms (-1)=w185) -> (notification=w187:string, timed out?=w183:bool)  [unwired: 2 in, 2 out]
    n99 = Equal?(x=w181, y=u16 2 ("Rec Mode")) -> (x = y?=w182:bool)
    n100 = Compound Arithmetic op=OR(invert w183, w182) -> (w184:bool)
    n101 = case shown="True" w184 {
      tunnel: w190 -> [_ w193]
      tunnel: w187 -> [_ w192]
      tunnel: w179 -> [_ w191]
      frame False {
      }
      frame True {
        n102 = call <vilib>:"Bind Controls to SmartDashboard.vi"("RPC ref"=w191, "Bound Control Refs"=w193, "Server IP Address"=w192) -> ()  [unwired: 9 in]
      }
    }
  }
  n103 = vi-ref "Playback Controls.vi"() -> (w64:refnum<vi>)
  n104 = property class="VI"() -> ("Panel"=w66:refnum<vi>)  [unwired: 2 in, 2 out]
  n105 = property class="Pnl"(reference=w66) -> ("Panes[]"=w67:refnum<vi>[])  [unwired: 1 in, 2 out]
  n106 = Index Array(array=w67) -> (element=w65:refnum<vi>)  [unwired: 1 in]
  n107 = control-ref of="Test Tree"() -> (w68:refnum<vi>)
  n108 = while {
    tunnel: [w203] -> _
    tunnel: w68 -> [w202]
    tunnel: w64 -> [w201]
    tunnel: w63 -> [w200]
    tunnel: w62 -> [_]
    tunnel: w58 -> [w199]
    tunnel: w25 -> [w198]
    tunnel: w23 -> [w197]
    shift-right: [w196] -> _
    shift-left: _ -> [w195]
    tunnel: w17 -> [w194]
    i -> [w203]
    stop <- FALSE stop-if-true
    n109 = event shown="[0] Timeout" {
      selector: w200 -> [_ _ _ _ _ _ _ _ _ _ _ _ _ _ _ _ _ _ _ _ _]
      dyn-events: [_ _ _ _ _ _ _ _ _ _ _ _ _ _ _ _ w463 _ _ _ _] -> _
      timeout: u32 60 ("milliseconds to wait") -> [_ _ _ _ _ _ _ _ _ _ _ _ _ _ _ _ _ _ _ _ _]
      tunnel: w202 -> [w215 _ _ _ _ _ _ _ _ _ _ _ _ _ _ _ _ _ _ _ _]
      tunnel: "Test Tree" -> [_ _ _ _ _ _ _ _ _ _ _ w430 w438 w440 w444 w452 _ _ _ _ _]
      tunnel: w201 -> [_ _ _ _ _ _ _ _ _ _ _ _ _ _ _ _ w465 _ w483 _ _]
      tunnel: w199 -> [_ _ _ _ _ _ _ _ _ _ _ _ _ _ _ _ w461 _ _ _ _]
      tunnel: w198 -> [_ _ _ _ _ _ _ _ _ _ _ _ _ _ _ _ w459 _ _ _ _]
      tunnel: w197 -> [w210 _ _ _ _ _ w381 _ _ _ _ _ _ _ _ _ _ _ _ _ _]
      tunnel: [w209 w258 w360 w365 w374 w378 w379 w388 w398 w405 w417 w429 w436 w439 w443 w451 w458 w478 w480 w484 w497] -> w196
      tunnel: w195 -> [w209 w258 w360 w365 w374 w378 w379 _ _ w405 w417 w429 w436 w439 w443 w451 w458 w478 w480 w484 w497]
      tunnel: w194 -> [w207 _ _ _ _ _ _ _ _ _ _ _ _ _ _ _ _ _ _ _ _]
      event Timeout {
        n110 = event-data() -> ()  [unwired: 1 in, 1 out]
        n111 = local read "Mode"() -> (w212:T4)
        n112 = case shown="\"Test\"" "Dashboard Tab" {
          tunnel: w215 -> [_ _ w231 _ _]
          tunnel: "TestMode/Automatic/" ("Name Pattern") -> [_ _ w230 _ _]
          tunnel: T22 [{"Operation"=enum."Clear", "Color Box"=14013909}, {"Operation"=enum."Clear", "Color Box"=14013909}, {"Operation"=enum."Clear", "Color Box"=14013909}, {"Operation"=enum."Clear", "Color Box"=14013909}, {"Operation"=enum."Update", "Color Box"=14013909}, {"Operation"=enum."Update", "Color Box"=16777215}, {"Operation"=enum."Clear", "Color Box"=14013909}, {"Operation"=enum."Clear", "Color Box"=14013909}, {"Operation"=enum."Clear", "Color Box"=14013909}] -> [_ _ w223 _ w251]
          tunnel: w212 -> [_ _ w222 _ w250]
          tunnel: u32[] [15790320, 15790320, 15790320, 15790320, 16777215, 16777215, 15790320, 15790320, 15790320] -> [_ _ _ _ w256]
          tunnel: w210 -> [_ _ _ _ w244]
          tunnel: w207 -> [_ w217 _ _ _]
          frame "Custom", Default {
          }
          frame "Basic" {
            n113 = call <vilib>:"WPI_DashboardUpdateNames.vi"("Controls on Tab"=w217) -> ()  [unwired: 11 in]
          }
          frame "Test" {
            w229 = -2 ("Active Item:Row Number")
            n114 = Index Array(array=w223, index=w222) -> (element=w224:T25)
            n115 = Unbundle(w224) -> ("Operation"=w225:enum16{"Update", "Clear"}, "Color Box"=w226:u32)
            n116 = call <vilib>:"NT Read String.vi"("Name"="TestMode/TestName") -> ("String"=w220:string)  [unwired: 9 in, 1 out]
            n117 = call <vilib>:"NT Read and Format Entries as Tree.vi"("Operation"=w225, "Name Pattern"=w230, "Tree Refnum"=w231) -> ()  [unwired: 7 in, 2 out]
            n118 = case shown="\"\"" w220 {
              tunnel: "TestMode/TestProgress" ("Name") -> [w233 _]
              tunnel: "TestMode/TestProgressText" ("Name") -> [w232 _]
              frame Default {
                n119 = call <vilib>:"NT Read Number.vi"("Name"=w233) -> ("Numeric"=w234:dbl)  [unwired: 9 in, 1 out]
                n120 = call <vilib>:"NT Read String.vi"("Name"=w232) -> ("String"=w235:string)  [unwired: 9 in, 1 out]
                n121 = Bundle("Numeric"=w234, "String"=w235) -> (→"Progress":cluster{"Numeric":dbl, "String":string})  [unwired: 1 in]
              }
              frame "" {
                n122 = property on="Progress" class="Clust (strict)"("Visible"=FALSE) -> ()  [unwired: 2 in, 2 out]
                n123 = local write "Test Name"(u16 0) -> ()
              }
            }
            n124 = property on="Test Tree" class="Tree (strict)"("Active Item Row Number"=w229, "ActiveColNum"=w229, "CellBG"=w226, "Active Item Row Number"=-1 ("Active Item:Row Number"), "CellBG"=u32 5789784 ("Color Box")) -> ()  [unwired: 2 in, 2 out]
          }
          frame "Variables" {
            w241 = string[] ["CameraPublisher", "Usage", "DB"]  # Items to initially close
            n125 = First Call?() -> (First Call?: T/F=w242:bool)
            n126 = control-ref of="Tree"() -> (w243:refnum<vi>)
            n127 = Select(t=w241, s=w242, f=string[] []) -> (s? t:f=w239:string[])
            n128 = call <vilib>:"NT Read and Format Entries as Tree.vi"("Tags to  Close"=w239, "Tree Refnum"=w243) -> ()  [unwired: 8 in, 2 out]
          }
          frame "Commands" {
            w252 = u32 5789784 ("Color Box")
            w253 = T26 {"Row"=-1, "Column"=-2} ("Active Cell:Active Cell")
            w255 = T26 {"Row"=-2, "Column"=-2} ("Active Cell:Active Cell")
            n129 = Index Array(array=w256, index=w250) -> (element=w254:u32)
            n130 = Index Array(array=w251, index=w250) -> (element=w249:T25)
            n131 = Unbundle(w249) -> ("Operation"=w248:enum16{"Update", "Clear"})  [unwired: 1 out]
            n132 = local read "Command Selection"() -> (w247:i32)
            n133 = property on="Command Selection" class="MCListbox (strict)"("ActiveCell"=w255, "CellBG"=w254, "ActiveCell"=w253, "CellBG"=w252) -> ()  [unwired: 2 in, 2 out]
            n134 = call <vilib>:"WPI_DashboardUpdate RPC Info.vi"("Operation"=w248) -> ("update"=w246:bool, "commands"=w245:string[][])  [unwired: 9 in]
            n135 = property on="Command Selection" class="MCListbox (strict)"("ItemNames"=w245) -> ()  [unwired: 2 in, 2 out]
            n136 = property on="Command Params" class="Tbl (strict)"("Active Cell"=w255, "Cell BG Color"=w254, "Active Cell"=w253, "Cell BG Color"=w252) -> ()  [unwired: 2 in, 2 out]
            n137 = call <vilib>:"WPI_DashboardUpdate Command Params.vi"("Update"=w246, "NewVal"=w247, "Commands"=w245, "Param Tbl"=w244) -> ()  [unwired: 7 in, 1 out]
          }
        }
        n138 = call <vilib>:"Connextion Info.vi"() -> ("Connected"=→"NT Connection":bool)  [unwired: 10 in, 1 out]
      }
      event "Test Tree": Value Change {
        # "Show appropriate\ncontrols"
        n139 = event-data() -> ("CtlRef"=w261:refnum<vi>, "NewVal"=w259:string)  [unwired: 1 in]
        n140 = call <vilib>:"WPI_UtilitiesGetTreeIOName.vi"("NewVal"=w259, "TreeControl in"=w261) -> ("I/O Name"=w262:string)  [unwired: 9 in]
        n141 = case shown="\"Camera\"" w262 {
          selector: w262 -> [_ w269 _ w291 w300 _]
          tunnel: w259 -> [_ _ w288 w290 _ w307]
          tunnel: cluster{string[]}[] [{["640x480", "320x240", "160x120"]}, {["Auto", "Fixed indoor", "Fixed outdoor 1", "Fixed outdoor 2", "Fixed fluorescent 1", "Fixed fluorescent 2", "Hold current"]}, {["Auto", "Flicker-free 50 Hz", "Flicker-free 60 Hz", "Hold current"]}, {["None", "Prioritize frame rate", "Prioritize image quality"]}, {["Monochrome", "Color"]}] -> [_ _ _ _ _ w306]
          frame Default {
            w264 = FALSE ("Visible")
            w263 = FALSE ("Visible")
            n142 = property on="Motor" class="Clust (strict)"("Visible"=w263) -> ()  [unwired: 2 in, 2 out]
            n143 = property on="Test Ring" class="Ring (strict)"("Visible"=w263) -> ()  [unwired: 2 in, 2 out]
            n144 = property on="Rev/Fwd" class="Clust (strict)"("Visible"=w264) -> ()  [unwired: 2 in, 2 out]
            n145 = property on="On/Off" class="Bool (strict)"("Visible"=w264) -> ()  [unwired: 2 in, 2 out]
            n146 = property on="Test Slider" class="Slide (strict)"("Visible"=w264) -> ()  [unwired: 2 in, 2 out]
          }
          frame "Analog Out", "Motor", "PWM" {
            w270 = FALSE ("Visible")
            n147 = case shown="\"Analog Out\"" w269 {
              tunnel: [1.0 ("Value") -1.0 ("Value") 0.0 ("Value")] -> w268
              tunnel: [255.0 ("Value") 1.0 ("Value") 5.0 ("Value")] -> w267
              tunnel: [128.0 ("Value") 0.0 ("Value") 0.0 ("Value")] -> w266
              tunnel: [64.0 ("Value") 0.5 ("Value") 1.0 ("Value")] -> w265
              frame "PWM" {
              }
              frame "Motor", Default {
              }
              frame "Analog Out" {
              }
            }
            n148 = property on="Motor" class="Clust (strict)"("Visible"=TRUE) -> ()  [unwired: 2 in, 2 out]
            n149 = property on="Value" class="Slide (strict)"("Value"=w266, "Scale.Minimum"=w268, "Scale.Maximum"=w267, "Scale.Increment"=w265) -> ()  [unwired: 2 in, 2 out]
            n150 = property on="On/Off" class="Bool (strict)"("Visible"=w270) -> ()  [unwired: 2 in, 2 out]
            n151 = property on="Test Slider" class="Slide (strict)"("Visible"=w270) -> ()  [unwired: 2 in, 2 out]
            n152 = property on="Test Ring" class="Ring (strict)"("Visible"=w270) -> ()  [unwired: 2 in, 2 out]
            n153 = property on="Rev/Fwd" class="Clust (strict)"("Visible"=w270) -> ()  [unwired: 2 in, 2 out]
          }
          frame "Servo" {
            w286 = FALSE ("Visible")
            n154 = call <vilib>:"NT Read Number.vi"("Name"=w288) -> ("Numeric"=w287:dbl)  [unwired: 9 in, 1 out]
            n155 = property on="Test Slider" class="Slide (strict)"("Visible"=TRUE, "Scale.Maximum"=170.0 ("Scale.Range:Maximum")) -> ()  [unwired: 2 in, 2 out]
            n156 = local write "Test Slider"(w287) -> ()
            n157 = property on="Motor" class="Clust (strict)"("Visible"=w286) -> ()  [unwired: 2 in, 2 out]
            n158 = property on="Rev/Fwd" class="Clust (strict)"("Visible"=w286) -> ()  [unwired: 2 in, 2 out]
            n159 = property on="On/Off" class="Bool (strict)"("Visible"=w286) -> ()  [unwired: 2 in, 2 out]
            n160 = property on="Test Ring" class="Ring (strict)"("Visible"=w286) -> ()  [unwired: 2 in, 2 out]
          }
          frame "Relay", "Solenoid" {
            w289 = FALSE ("Visible")
            n161 = property on="Motor" class="Clust (strict)"("Visible"=w289) -> ()  [unwired: 2 in, 2 out]
            n162 = property on="Test Slider" class="Slide (strict)"("Visible"=w289) -> ()  [unwired: 2 in, 2 out]
            n163 = Search and Replace String(input string=w290, search string="/Value  **", replace string="/Direction") -> (result string=w296:string)  [unwired: 5 in, 3 out]
            n164 = property on="Test Ring" class="Ring (strict)"("Visible"=w289) -> ()  [unwired: 2 in, 2 out]
            n165 = call <vilib>:"NT Read String.vi"("Name"=w296) -> ("String"=w294:string)  [unwired: 9 in, 1 out]
            n166 = Equal?(x="Both directions", y=w294) -> (x = y?=w292:bool)
            n167 = Not(x=w292) -> (.not. x?=w293:bool)
            n168 = property on="Rev/Fwd" class="Clust (strict)"("Visible"=w292) -> ()  [unwired: 2 in, 2 out]
            n169 = property on="On/Off" class="Bool (strict)"("Visible"=w293, "Caption.Text"=w291) -> ()  [unwired: 2 in, 2 out]
          }
          frame "Compressor", "Digital Out" {
            w299 = FALSE ("Visible")
            # "Get direction and finish"
            n170 = property on="Motor" class="Clust (strict)"("Visible"=w299) -> ()  [unwired: 2 in, 2 out]
            n171 = property on="Test Slider" class="Slide (strict)"("Visible"=w299) -> ()  [unwired: 2 in, 2 out]
            n172 = property on="Test Ring" class="Ring (strict)"("Visible"=w299) -> ()  [unwired: 2 in, 2 out]
            n173 = property on="On/Off" class="Bool (strict)"("Visible"=TRUE, "Caption.Text"=w300) -> ()  [unwired: 2 in, 2 out]
            n174 = property on="Rev/Fwd" class="Clust (strict)"("Visible"=FALSE) -> ()  [unwired: 2 in, 2 out]
          }
          frame "Camera" {
            n175 = call <vilib>:"Get Last Path Segment.vi"("String in"=w307) -> ("String out"=w308:string)  [unwired: 10 in]
            n176 = property on="On/Off" class="Bool (strict)"("Visible"=FALSE) -> ()  [unwired: 2 in, 2 out]
            n177 = property on="Motor" class="Clust (strict)"("Visible"=FALSE) -> ()  [unwired: 2 in, 2 out]
            n178 = property on="Rev/Fwd" class="Clust (strict)"("Visible"=FALSE) -> ()  [unwired: 2 in, 2 out]
            n179 = case shown="\"White Balance  **\"" w308 {
              tunnel: w307 -> [w314 w323 w332 w341 w350 _ w356]
              tunnel: w306 -> [w312 w320 w329 w338 w347 _ _]
              frame "Size  **" {
                n180 = Index Array(array=w312) -> (element=w311:cluster{string[]})  [unwired: 1 in]
                n181 = call <vilib>:"NT Read String.vi"("Name"=w314) -> ("String"=w313:string)  [unwired: 9 in, 1 out]
                n182 = Unbundle(w311) -> (w309:string[])
                n183 = Match First String(2:w309, 3:w313) -> (0:w310:i32)  [unwired: 1 out]
                n184 = property on="Test Ring" class="Ring (strict)"("Value"=w310, "Strings []"=w309) -> ()  [unwired: 2 in, 2 out]
                n185 = property on="Test Ring" class="Ring (strict)"("Visible"=TRUE) -> ()  [unwired: 2 in, 2 out]
                n186 = property on="Test Slider" class="Slide (strict)"("Visible"=FALSE) -> ()  [unwired: 2 in, 2 out]
              }
              frame "White Balance  **" {
                n187 = Index Array(array=w320, index=1) -> (element=w321:cluster{string[]})
                n188 = call <vilib>:"NT Read String.vi"("Name"=w323) -> ("String"=w322:string)  [unwired: 9 in, 1 out]
                n189 = Unbundle(w321) -> (w318:string[])
                n190 = Match First String(2:w318, 3:w322) -> (0:w317:i32)  [unwired: 1 out]
                n191 = property on="Test Ring" class="Ring (strict)"("Value"=w317, "Strings []"=w318) -> ()  [unwired: 2 in, 2 out]
                n192 = property on="Test Ring" class="Ring (strict)"("Visible"=TRUE) -> ()  [unwired: 2 in, 2 out]
                n193 = property on="Test Slider" class="Slide (strict)"("Visible"=FALSE) -> ()  [unwired: 2 in, 2 out]
              }
              frame "Exposure  **" {
                n194 = Index Array(array=w329, index=2) -> (element=w330:cluster{string[]})
                n195 = call <vilib>:"NT Read String.vi"("Name"=w332) -> ("String"=w331:string)  [unwired: 9 in, 1 out]
                n196 = Unbundle(w330) -> (w326:string[])
                n197 = Match First String(2:w326, 3:w331) -> (0:w327:i32)  [unwired: 1 out]
                n198 = property on="Test Ring" class="Ring (strict)"("Value"=w327, "Strings []"=w326) -> ()  [unwired: 2 in, 2 out]
                n199 = property on="Test Ring" class="Ring (strict)"("Visible"=TRUE) -> ()  [unwired: 2 in, 2 out]
                n200 = property on="Test Slider" class="Slide (strict)"("Visible"=FALSE) -> ()  [unwired: 2 in, 2 out]
              }
              frame "Exposure Priority  **" {
                n201 = Index Array(array=w338, index=3) -> (element=w339:cluster{string[]})
                n202 = call <vilib>:"NT Read String.vi"("Name"=w341) -> ("String"=w340:string)  [unwired: 9 in, 1 out]
                n203 = Unbundle(w339) -> (w335:string[])
                n204 = Match First String(2:w335, 3:w340) -> (0:w336:i32)  [unwired: 1 out]
                n205 = property on="Test Ring" class="Ring (strict)"("Value"=w336, "Strings []"=w335) -> ()  [unwired: 2 in, 2 out]
                n206 = property on="Test Ring" class="Ring (strict)"("Visible"=TRUE) -> ()  [unwired: 2 in, 2 out]
                n207 = property on="Test Slider" class="Slide (strict)"("Visible"=FALSE) -> ()  [unwired: 2 in, 2 out]
              }
              frame "Color Enable  **" {
                n208 = Index Array(array=w347, index=4) -> (element=w348:cluster{string[]})
                n209 = call <vilib>:"NT Read String.vi"("Name"=w350) -> ("String"=w349:string)  [unwired: 9 in, 1 out]
                n210 = Unbundle(w348) -> (w344:string[])
                n211 = Match First String(2:w344, 3:w349) -> (0:w345:i32)  [unwired: 1 out]
                n212 = property on="Test Ring" class="Ring (strict)"("Value"=w345, "Strings []"=w344) -> ()  [unwired: 2 in, 2 out]
                n213 = property on="Test Ring" class="Ring (strict)"("Visible"=TRUE) -> ()  [unwired: 2 in, 2 out]
                n214 = property on="Test Slider" class="Slide (strict)"("Visible"=FALSE) -> ()  [unwired: 2 in, 2 out]
              }
              frame Default {
                n215 = property on="Test Ring" class="Ring (strict)"("Visible"=FALSE) -> ()  [unwired: 2 in, 2 out]
                n216 = property on="Test Slider" class="Slide (strict)"("Visible"=FALSE) -> ()  [unwired: 2 in, 2 out]
              }
              frame "Brightness  **", "Color Level  **", "Compression  **", "FPS  **", "Sharpness  **" {
                n217 = call <vilib>:"NT Read Number.vi"("Name"=w356) -> ("Numeric"=w355:dbl)  [unwired: 9 in, 1 out]
                n218 = local write "Test Slider"(w355) -> ()
                n219 = property on="Test Slider" class="Slide (strict)"("Visible"=TRUE, "Scale.Maximum"=100.0 ("Scale.Range:Maximum")) -> ()  [unwired: 2 in, 2 out]
                n220 = property on="Test Ring" class="Ring (strict)"("Visible"=FALSE) -> ()  [unwired: 2 in, 2 out]
              }
            }
          }
        }
        n221 = property on="Progress" class="Clust (strict)"("Visible"=FALSE) -> ()  [unwired: 2 in, 2 out]
      }
      event "Test Name": Mouse Enter {
        # "Populate the ring with the list of tests"
        n222 = event-data() -> ()  [unwired: 1 in, 1 out]
        n223 = call <vilib>:"NT Read String Array.vi"("Name"="TestMode/TestList") -> ("String Array"=w364:string[])  [unwired: 9 in, 1 out]
        n224 = Build Array (concatenate)("Select the test to run...", w364) -> (w363:string[])
        n225 = property on="Test Name" class="Ring (strict)"("Strings []"=w363) -> ()  [unwired: 2 in, 2 out]
      }
      event "Test Name": Value Change {
        w366 = FALSE ("Visible")
        # "Tell the robot the test name to run"
        n226 = event-data() -> ("NewVal"=w370:u16)  [unwired: 1 in]
        n227 = property on="Test Name" class="Ring (strict)"() -> ("Strings []"=w371:string[])  [unwired: 2 in, 2 out]
        n228 = local write "Progress"(T7 {"Test Progress"=0, "Test Progress Text"=""} ("Progress")) -> ()
        n229 = Index Array(array=w371, index=w370) -> (element=w369:string)
        n230 = call <vilib>:"NT Write String.vi"("String"=w369, "Name"="TestMode/TestName") -> ()  [unwired: 9 in, 1 out]
        n231 = property on="Progress" class="Clust (strict)"("Visible"=TRUE) -> ()  [unwired: 2 in, 2 out]
        n232 = property on="Motor" class="Clust (strict)"("Visible"=w366) -> ()  [unwired: 2 in, 2 out]
        n233 = property on="Test Slider" class="Slide (strict)"("Visible"=w366) -> ()  [unwired: 2 in, 2 out]
        n234 = property on="On/Off" class="Bool (strict)"("Visible"=w366) -> ()  [unwired: 2 in, 2 out]
        n235 = property on="Rev/Fwd" class="Clust (strict)"("Visible"=w366) -> ()  [unwired: 2 in, 2 out]
        n236 = property on="Test Ring" class="Ring (strict)"("Visible"=w366) -> ()  [unwired: 2 in, 2 out]
      }
      event "Select Auto": Mouse Enter {
        # "Populate the combo box with the list of autonomous options"
        n237 = event-data() -> ()  [unwired: 1 in, 1 out]
        n238 = call <vilib>:"NT Read String Array.vi"("Name"="Auto List") -> ("String Array"=w373:string[])  [unwired: 9 in, 1 out]
        n239 = property on="Select Auto" class="CmbBox"("Strings[]"=w373) -> ()  [unwired: 2 in, 2 out]
      }
      event "Select Auto": Value Change {
        # "User modified the Auto Selection. Write to NT variable so robot knows."
        n240 = event-data() -> ("NewVal"=w376:string)  [unwired: 1 in]
        n241 = call <vilib>:"NT Write String.vi"("String"=w376, "Name"="Auto Selector") -> ()  [unwired: 9 in, 1 out]
      }
      event "Command Selection": Value Change {
        # "Get the params and show in table"
        n242 = event-data() -> ("NewVal"=w382:i32)  [unwired: 1 in]
        n243 = property on="Command Selection" class="MCListbox (strict)"() -> ("ItemNames"=w380:string[][])  [unwired: 2 in, 2 out]
        n244 = call <vilib>:"WPI_DashboardUpdate Command Params.vi"("NewVal"=w382, "Commands"=w380, "Param Tbl"=w381) -> ()  [unwired: 8 in, 1 out]
      }
      event "Execute Command": Value Change {
        # "Started one, Unique ID holds\nresponse"
        n245 = event-data() -> ()  [unwired: 1 in, 1 out]
        n246 = property on="Command Selection" class="MCListbox (strict)"() -> ("ItemNames"=w393:string[][])  [unwired: 2 in, 2 out]
        n247 = Index Array(array=w393, index (row)="Command Selection", index (col)=0) -> (element=w391:string)
        n248 = call <vilib>:"Invoke Commands.vi"("Command Params"="Command Params", "Function Name"=w391) -> ("Params"=w387:u8, "Started"=w386:bool)  [unwired: 7 in, 1 out]
        n249 = Array Subset(array="Command Params", length (row)=w387) -> (w388:string[][])  [unwired: 3 in]
        n250 = Select(t="Executing" ("Cmd Status"), s=w386, f="" ("Cmd Status")) -> (s? t:f=→"Cmd Status":string)
      }
      event "Command Selection": Double Click {
        n251 = event-data() -> ("Row"=w401:i32)  [unwired: 1 in]
        n252 = property on="Command Selection" class="MCListbox (strict)"() -> ("ItemNames"=w404:string[][])  [unwired: 2 in, 2 out]
        n253 = local read "Command Params"() -> (w400:string[][])
        n254 = Index Array(array=w404, index (row)=w401, index (col)=0) -> (element=w402:string)
        n255 = call <vilib>:"Invoke Commands.vi"("Command Params"=w400, "Function Name"=w402) -> ("Params"=w399:u8, "Started"=w394:bool)  [unwired: 7 in, 1 out]
        n256 = Array Subset(array=w400, length (row)=w399) -> (w398:string[][])  [unwired: 3 in]
        n257 = Select(t="Executing" ("Cmd Status"), s=w394, f="" ("Cmd Status")) -> (s? t:f=w395:string)
        n258 = local write "Cmd Status"(w395) -> ()
      }
      event "CheckList": Double Click {
        # "Shift clears all"
        # "Update symbols on the listbox"
        n259 = event-data() -> ("PlatMods.Shift"=w406:bool, "Row"=w408:i32)  [unwired: 1 in]
        n260 = case shown="True" w406 {
          tunnel: w408 -> [w412 _]
          tunnel: 1 -> [w411 _]
          frame False {
            n261 = property on="CheckList" class="LstBox (strict)"() -> ("Item Symbols"=w410:i32[])  [unwired: 2 in, 2 out]
            n262 = Replace Array Subset(array=w410, new element=w411, index=w412) -> (w409:i32[])
            n263 = property on="CheckList" class="LstBox (strict)"("Item Symbols"=w409) -> ()  [unwired: 2 in, 2 out]
          }
          frame True {
            w413 = 0 ("Top Row")
            n264 = property on="CheckList" class="LstBox (strict)"() -> ("Number of Rows"=w415:u32)  [unwired: 2 in, 2 out]
            n265 = Initialize Array(0, w415) -> (w414:i32[])
            n266 = property on="CheckList" class="LstBox (strict)"("Top Row"=w413, "Value"=w413, "Item Symbols"=w414) -> ()  [unwired: 2 in, 2 out]
          }
        }
      }
      event "CheckList": Key Down {
        # "Update symbols on the listbox\nLeft and right keys check and uncheck"
        n267 = event-data() -> ("VKey"=w419:T23)  [unwired: 1 in]
        n268 = case shown="\"Left\", \"Right\"" w419 {
          selector: w419 -> [w424 _]
          tunnel: eventvkey."Left" ("VKey") -> [w422 _]
          frame "Left", "Right" {
            n269 = Equal?(x=w422, y=w424) -> (x = y?=w423:bool)
            n270 = Select(t=0, s=w423, f=1) -> (s? t:f=w425:i32)
            n271 = property on="CheckList" class="LstBox (strict)"() -> ("Item Symbols"=w428:i32[])  [unwired: 2 in, 2 out]
            n272 = Replace Array Subset(array=w428, new element=w425, index="CheckList") -> (w427:i32[])
            n273 = property on="CheckList" class="LstBox (strict)"("Item Symbols"=w427) -> ()  [unwired: 2 in, 2 out]
          }
          frame Default {
          }
        }
      }
      event "Motor.Enable": Value Change {
        # "When the test mode otor enable helper is set, update that\ntree row item's value"
        n274 = event-data() -> ("NewVal"=w434:bool)  [unwired: 1 in]
        n275 = Unbundle("Motor") -> ("Value"=w433:dbl)  [unwired: 1 out]
        n276 = Select(t=w433, s=w434, f=0.0) -> (s? t:f=w431:dbl)
        n277 = call <vilib>:"NT Write Number.vi"("Numeric"=w431, "Name"=w430) -> ()  [unwired: 9 in, 1 out]
      }
      event "Test Slider": Value Change {
        # "When the test mode slider helper is set, update that\ntree row item's value"
        n278 = event-data() -> ("NewVal"=w437:dbl)  [unwired: 1 in]
        n279 = call <vilib>:"NT Write Number.vi"("Numeric"=w437, "Name"=w438) -> ()  [unwired: 9 in, 1 out]
      }
      event "On/Off": Value Change {
        # "When the test mode on/off helper value is set, update that\ntree row item's value"
        n280 = event-data() -> ("NewVal"=w442:bool)  [unwired: 1 in]
        n281 = Boolean To (0,1)(Boolean=w442) -> (0, 1=w441:i16)
        n282 = call <vilib>:"NT Write Number.vi"("Numeric"=w441, "Name"=w440) -> ()  [unwired: 9 in, 1 out]
      }
      event "Rev/Fwd": Value Change {
        # "When the test mode helper value for relays is set, update that\ntree row item's value"
        n283 = event-data() -> ("NewVal.Forward"=w450:bool, "NewVal.Reverse"=w449:bool)  [unwired: 1 in]
        n284 = Boolean To (0,1)(Boolean=w450) -> (0, 1=w446:i16)
        n285 = Boolean To (0,1)(Boolean=w449) -> (0, 1=w448:i16)
        n286 = Negate(x=w448) -> (-x=w447:i16)
        n287 = Add(x=w446, y=w447) -> (x+y=w445:i16)
        n288 = call <vilib>:"NT Write Number.vi"("Numeric"=w445, "Name"=w444) -> ()  [unwired: 9 in, 1 out]
      }
      event "Test Ring": Value Change {
        # "When a test mode helper value is selected from the ring,\nset the tree item's variable to the string value"
        n289 = event-data() -> ("NewVal"=w454:u16)  [unwired: 1 in]
        n290 = property on="Test Ring" class="Ring (strict)"() -> ("Strings []"=w455:string[])  [unwired: 2 in, 2 out]
        n291 = Index Array(array=w455, index=w454) -> (element=w453:string)
        n292 = call <vilib>:"NT Write String.vi"("String"=w453, "Name"=w452) -> ()  [unwired: 9 in, 1 out]
      }
      event "Rec Mode": Value Change {
        # "Update globals for recording mode and path to read log from.\nClear when logging and let NetworkTables set path for vision to\nuse."
        n293 = event-data() -> ("NewVal"=w466:enum32{"Stop", "Record", "Playback"})  [unwired: 1 in]
        n294 = global write "WPI_DashboardLogging Global.vi" "Logging Filename"(path "") -> ()
        n295 = global write "WPI_DashboardLogging Global.vi" "Recording"(w466) -> ()
        n296 = case shown="\"Playback\"" w466 {
          tunnel: w465 -> [_ w468 w477]
          tunnel: [_ _ w476] -> w463
          tunnel: [_ _ w475] -> _
          tunnel: w461 -> [_ _ w473]
          tunnel: cluster{i32, i32} {-250, 170} -> [_ _ w472]
          tunnel: [_ _ T24 {"Image Size"=TRUE, "Image Type"=TRUE, "Pixel Value"=TRUE, "ROI Information"=TRUE, "Zoom Factor"=FALSE} ("Image Information Shown:All Elements")] -> w456
          tunnel: [_ _ TRUE ("Zoom Factor")] -> w457
          tunnel: w459 -> [_ _ w469]
          frame Default {
          }
          frame "Stop", "Record" {
            # "Place Window too"
            n297 = invoke class="VI" method="FP.Close"(reference=w468) -> (reference out=w467:refnum<vi>)  [unwired: 2 in, 2 out]
            n298 = invoke class="VI" method="Abort VI"(reference=w467) -> ()  [unwired: 2 in, 3 out]
          }
          frame "Playback" {
            n299 = call "Open Playback Panel.vi"("Offset"=w472, "DB VI Ref"=w473, "Playback in"=w477) -> ("Playback out"=w474:refnum<vi>)  [unwired: 8 in]
            n300 = register-events(w474, w469) -> (reference out=w476:refnum<event-registration>, error out=w475:errorcluster)  [unwired: 2 in]
          }
        }
        n301 = property on="Camera Image Right" class="ImageControl"("Image Information Shown"=w456, "Image Information Visible"=w457) -> ()  [unwired: 2 in, 2 out]
        n302 = property on="Camera Image" class="ImageControl"("Image Information Shown"=w456, "Image Information Visible"=w457) -> ()  [unwired: 2 in, 2 out]
        n303 = call <vilib>:"WPI_DashboardNT Log FieldName Cache.vi"("Operation"=enum16{"Lookup/Add", "Index", "Clear"}."Clear") -> ()  [unwired: 8 in, 3 out]
      }
      event Panel Close {
        w479 = enum32{"Stop", "Record", "Playback"}."Stop" ("Rec Mode")
        # "Playback window has been closed, abort"
        n304 = event-data() -> ()  [unwired: 1 in, 4 out]
        n305 = local write "Rec Mode"(w479) -> ()
        n306 = global write "WPI_DashboardLogging Global.vi" "Recording"(w479) -> ()
      }
      event Panel Close {
        # "Abort playback window and ourself"
        n307 = event-data() -> ()  [unwired: 1 in, 4 out]
        n308 = invoke class="VI" method="FP.Close"(reference=w483) -> (reference out=w482:refnum<vi>)  [unwired: 2 in, 2 out]
        n309 = invoke class="VI" method="Abort VI"(reference=w482) -> (error out=w481:errorcluster)  [unwired: 2 in, 2 out]
        n310 = invoke class="VI" method="Abort VI"(error in=w481) -> ()  [unwired: 2 in, 3 out]
      }
      event User Event {
        n311 = event-data() -> ("IDs"=w490:cluster{"RPC field ID":u16, "Unique ID":u16}, "String"=w489:string)  [unwired: 1 in]
        n312 = Bundle("IDs"=w490, "String"=w489) -> (w488:T10)  [unwired: 1 in]
        n313 = call <vilib>:"Retrieve RPC Response.vi"("RPC Response"=w488) -> ("Output"=w486:string[][])  [unwired: 10 in]
        n314 = Build Array (concatenate)(w484, w486) -> (w485:string[][])
        n315 = local write "Command Params"(w485) -> ()
        n316 = local write "Cmd Status"("" ("Cmd Status")) -> ()
      }
      event "Tree": Double Click {
        n317 = event-data() -> ("PlatMods"=w496:T27, "Tag"=w493:string)  [unwired: 1 in]
        n318 = Unbundle(w496) -> ("Shift"=w495:bool)  [unwired: 4 out]
        n319 = String Subset(string=w493, length (rest)=1 ("length (rest)")) -> (substring=w492:string)  [unwired: 1 in]
        n320 = Not(x=w495) -> (.not. x?=w494:bool)
        n321 = case shown="\"/\"" w492 {
          tunnel: w493 -> [_ w499]
          tunnel: w494 -> [_ w498]
          frame Default {
          }
          frame "/" {
            n322 = call <vilib>:"NT Update Persistence.vi"("Persistence"=w498, "Name"=w499) -> ()  [unwired: 9 in, 1 out]
          }
        }
      }
    }
  }
  n323 = while {
    tunnel: w65 -> [w501]
    i -> [w504]
    stop <- FALSE stop-if-true
    n324 = Wait (ms)(milliseconds to wait=u32 100) -> ()  [unwired: 1 out]
    n325 = case shown="\"Playback\"" "Rec Mode" {
      tunnel: w504 -> [_ _ w519]
      tunnel: [u32 2829099 ("Base Color") u32 11141120 ("Target Color") w508] -> w500
      frame "Stop", Default {
        # "Reset the color, extra updates don't cost much"
      }
      frame "Record" {
      }
      frame "Playback" {
        # "Playback"
        n326 = Quotient & Remainder(x=w519, y=u32 50 ("milliseconds to wait")) -> (x-y*floor(x/y)=w515:u32)  [unwired: 1 out]
        n327 = Divide(x=w515, y=u32 50 ("milliseconds to wait")) -> (x/y=w512:dbl)
        n328 = Multiply(x=6.283185307179586, y=w512) -> (x*y=w517:dbl)
        n329 = Sine(x=w517) -> (sin(x)=w516:dbl)
        n330 = Absolute Value(x=w516) -> (abs(x)=w509:dbl)
        n331 = call "Interpolate RGB Color.vi"("Proportion"=w509, "Target Color"=u32 30976, "Base Color"=u32 2829099) -> ("Result Color"=w508:u32)  [unwired: 8 in]
      }
    }
    n332 = property class="Pane"(reference=w501, "PaneColor"=w500) -> ()  [unwired: 1 in, 2 out]
  }
  n333 = local write "Dashboard Tab"(T2."Drive" ("Dashboard Tab")) -> ()
  n334 = property on="On/Off" class="Bool (strict)"("Visible"=w36) -> ()  [unwired: 2 in, 2 out]
  n335 = property on="Motor" class="Clust (strict)"("Visible"=w36) -> ()  [unwired: 2 in, 2 out]
  n336 = property on="Progress" class="Clust (strict)"("Visible"=w36) -> ()  [unwired: 2 in, 2 out]
  n337 = property on="Test Ring" class="Ring (strict)"("Visible"=w36) -> ()  [unwired: 2 in, 2 out]
  n338 = property on="Rev/Fwd" class="Clust (strict)"("Visible"=w36) -> ()  [unwired: 2 in, 2 out]
  n339 = while {
    tunnel: u16 1741 ("timeout ms (25000)") -> [w521]
    stop <- FALSE stop-if-true
    n340 = TCP Create Listener(10:w521) -> (0:w520:errorcluster, 3:w522:refnum<k5>)  [unwired: 4 in, 1 out]
    n341 = case shown="No Error" w520 {
      selector: w520 -> [w524 _]
      tunnel: w522 -> [w525 _]
      frame No Error {
        n342 = while {
          tunnel: w525 -> [w528]
          tunnel: w524 -> [w527]
          stop <- FALSE stop-if-true
          n343 = TCP Wait On Listener(8:w527, 11:w528) -> (0:w529:errorcluster, 4:w530:refnum<k5>)  [unwired: 2 in, 3 out]
          n344 = local write "TCP"(w530) -> ()
          n345 = case shown="No Error" w529 {
            frame No Error {
            }
            frame Error {
              n346 = Wait (ms)(milliseconds to wait=u32 1000) -> ()  [unwired: 1 out]
            }
          }
        }
      }
      frame Error {
        n347 = Wait (ms)(milliseconds to wait=u32 1000) -> ()  [unwired: 1 out]
      }
    }
  }
  n348 = local write "Command Selection"(u16 0 ("milliseconds to wait")) -> ()
  n349 = local write "Command Params"(string[][] [] ("Command Params")) -> ()
  n350 = global write "WPI_DashboardLogging Global.vi" "Recording"(w59) -> ()
  n351 = local write "Rec Mode"(w59) -> ()
  n352 = call <vilib>:"NT Write String.vi"("String"="Select Auto", "Name"="Auto Selector") -> ()  [unwired: 9 in, 1 out]
